vi "GV frame counter.vi"() -> ()   [LabVIEW 2017]
panel:
  out "Frame counter":u8
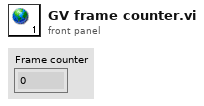
[diagram p1: front panel]
diagram:
